vi "Get Scanner.vi"(8 "error in (no error)":errorcluster, 11 "Function Generator in":refnum<class "Function Generator.lvclass">) -> (0 "error out":errorcluster, 2 "Default Scanner out":refnum<class "Scanner.lvclass">)   [LabVIEW 2017, in "Function Generator.lvclass"]
doc: "(Dynamic) Returns the default Scanner object that scans over this Scannable. (Note that a Scannable may have multiple Scanners associated with it.) A Scanner is an analogue to an Iterator class in other languages."
uses:
  Function Generator.lvclass
  Scanners/Scanner/Scanner.lvclass
  Scanners/Function Gen Scan/Function Gen Scan.lvclass
  C:/LabVIEW-programs-dev/Scanners/Scanner/Scanner.lvclass
  Utility Classes/Scannable/Scannable.lvclass
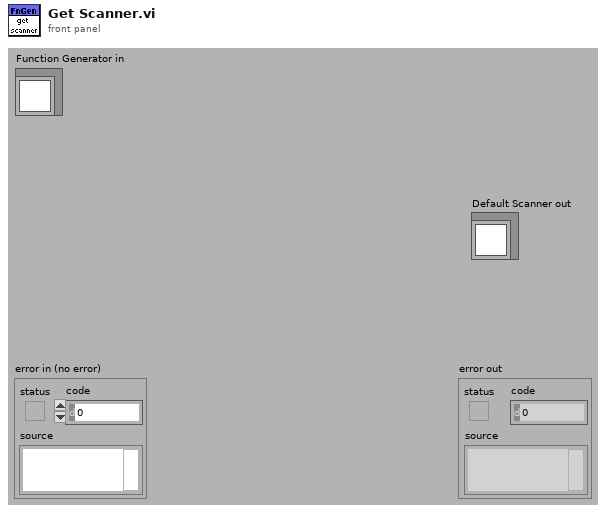
[diagram p1: front panel]
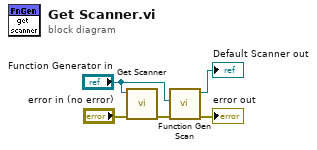
[diagram p0: block diagram]
diagram:
  n1 = call-parent "Get Scanner.vi"("error in (no error)"="error in (no error)", "Scannable in"="Function Generator in") -> ("error out"=w3:errorcluster)  [unwired: 9 out]
  n2 = call "Function Gen Scan.vi"("error in (no error)"=w3, "Function Generator.lvclass"="Function Generator in") -> ("error out"=→"error out":errorcluster, "Function Gen Scan out"=→"Default Scanner out":refnum<class "Function Gen Scan.lvclass">)  [unwired: 8 out]
